vi "lab2_new_p1_2.vi"() -> ()   [LabVIEW 2021]
panel:
  in  "n":i64
  in  "x":dbl
  out "N!":dbl
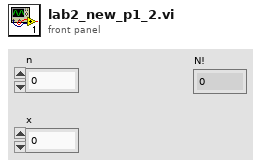
[diagram p1: front panel]
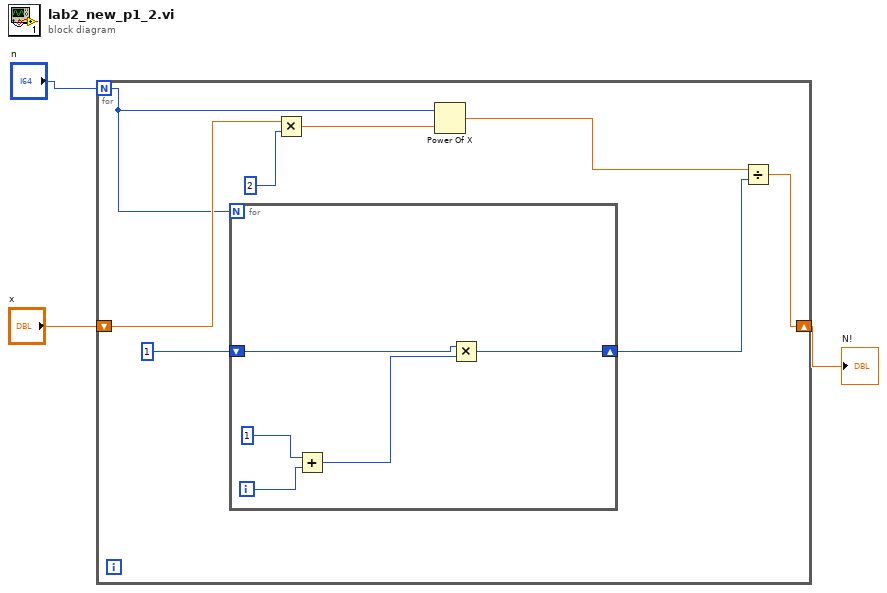
[diagram p0: block diagram]
diagram:
  n1 = for {
    N: "n" -> [w7]
    shift-right: [w5] -> w3
    shift-left: "x" -> [w8]
    n2 = for {
      N: w7 -> [_]
      shift-right: [w12] -> w4
      shift-left: 1 -> [w13]
      i -> [w15]
      n3 = Add(x=1, y=w15) -> (x+y=w14:i32)
      n4 = Multiply(x=w13, y=w14) -> (x*y=w12:i32)
    }
    n5 = Multiply(x=w8, y=2) -> (x*y=w9:dbl)
    n6 = Power Of X(1:w9, 2:w7) -> (0:w6:dbl)
    n7 = Divide(x=w6, y=w4) -> (x/y=w5:dbl)
  }
  "N!" <- w3
